vi "Copy Builds To NIVS Dir.vi"(5 "Files Generated by Build":path[](array[path]), 6 "Top Level/Always Included VIs":path[](array[path]), 7 "Destination Path":path, 8 "error in (no error)":errorcluster, 9 "Target Name":string, 10 "Build Specification Name":string, 11 "Project Path":path) -> (0 "error out":errorcluster)   [LabVIEW 2013]
uses:
  <vilib>/Utility/sysdir.llb/System Directory Type.ctl
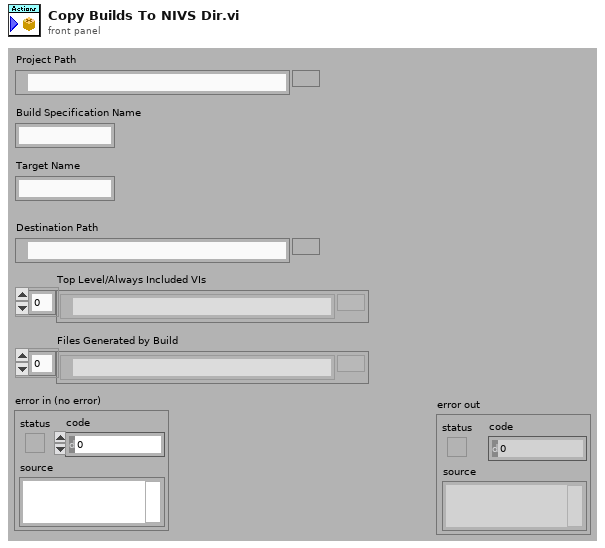
[diagram p1: front panel]
types:
  T1 = typedef "System Directory Type.ctl" = i32
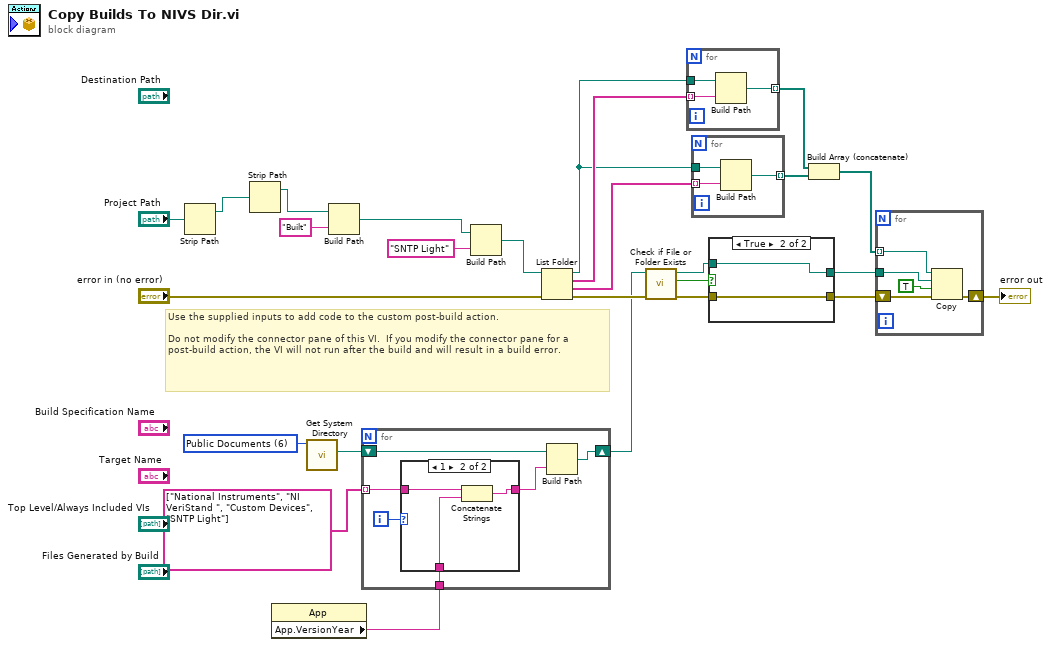
[diagram p0: block diagram]
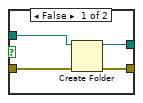
[diagram p3: hidden frame]
diagram:
  w9 = T1 6 items=["User Home"=0, "User Desktop"=1, "User Documents"=2, "User Application Data"=3, "User Preferences"=4, "User Temporary"=5, "Public Documents"=6, "Public Application Data"=7, "Public Preferences"=8, "Public Cache"=13, "System Core Libraries"=9, "System Installed Libraries"=10, "Application Files"=11, "Boot Volume Root"=12] ("system directory type")
  # "Use the supplied inputs to add code to the custom post-build action.\n\nDo not modify the connector pane of this VI.  If you modify the connector pane for a post-build action, the VI will not run after the build and will result in a build error."
  n1 = Strip Path(path="Project Path") -> (stripped path=w2:path)  [unwired: 1 out]
  n2 = Strip Path(path=w2) -> (stripped path=w1:path)  [unwired: 1 out]
  n3 = property class="App"() -> ("App.VersionYear"=w5:string)  [unwired: 2 in, 2 out]
  n4 = call <vilib>:"Get System Directory.vi"("system directory type"=w9) -> ("system directory"=w8:path)  [unwired: 10 in]
  n5 = Build Path(base path=w1, name or relative path="Built") -> (appended path=w4:path)
  n6 = for {
    shift-right: [w31] -> w6
    shift-left: w8 -> [w32]
    tunnel: string[] ["National Instruments", "NI VeriStand ", "Custom Devices", "SNTP Light"] -> [w28] mode=indexing
    tunnel: w5 -> [w27]
    i -> [w30]
    n7 = case shown="1" w30 {
      tunnel: [w33 w35] -> w29
      tunnel: w28 -> [w33 w36]
      tunnel: w27 -> [_ w34]
      frame Default {
      }
      frame 1 {
        n8 = Concatenate Strings(w36, w34) -> (w35:string)
      }
    }
    n9 = Build Path(base path=w32, name or relative path=w29) -> (appended path=w31:path)
  }
  n10 = Build Path(base path=w4, name or relative path="SNTP Light") -> (appended path=w12:path)
  n11 = List Folder(path=w12, error in="error in (no error)") -> (path out=w14:path, filenames=w26:string[], folder names=w15:string[], error out=w10:errorcluster)  [unwired: 2 in]
  n12 = call <vilib>:"Check if File or Folder Exists.vi"("error in (no error)"=w10, "path"=w6) -> ("error out"=w18:errorcluster, "file or folder exists?"=w20:bool, "dup path"=w19:path)  [unwired: 7 in]
  n13 = for {
    tunnel: w26 -> [w38] mode=indexing
    tunnel: w14 -> [w39]
    tunnel: [w37] -> w25 mode=indexing
    n14 = Build Path(base path=w39, name or relative path=w38) -> (appended path=w37:path)
  }
  n15 = for {
    tunnel: w15 -> [w41] mode=indexing
    tunnel: w14 -> [w42]
    tunnel: [w40] -> w13 mode=indexing
    n16 = Build Path(base path=w42, name or relative path=w41) -> (appended path=w40:path)
  }
  n17 = case shown="True" w20 {
    tunnel: w19 -> [w46 w48]
    tunnel: w18 -> [w45 w47]
    tunnel: [w44 w48] -> w17
    tunnel: [w43 w47] -> w16
    frame False {
      n18 = Create Folder(path (use dialog)=w46, error in=w45) -> (created path=w44:path, error out=w43:errorcluster)  [unwired: 1 in, 1 out]
    }
    frame True {
    }
  }
  n19 = Build Array (concatenate)(w25, w13) -> (w24:path[])
  n20 = for {
    tunnel: w24 -> [w50] mode=indexing
    shift-right: [w51] -> w3
    shift-left: w16 -> [w52]
    tunnel: w17 -> [w49]
    n21 = Copy(8:w52, 9:TRUE ("overwrite (F)"), 10:w49, 11:w50) -> (0:w51:errorcluster)  [unwired: 1 in, 2 out]
  }
  "error out" <- w3
